vi "Set - Scalar - Complex.vi"(8 "error in":errorcluster, 9 "value":cdb, 10 "variable name":string, 11 "pipe in":T1) -> (0 "error out":errorcluster, 3 "pipe out":T1)   [LabVIEW 2013, in "GOLPI library.lvlib"]
uses:
  GOLPI library.lvlib
  LV Process.lvlibp/Pipe Handle.ctl
  Globals.vi
  LV Process.lvlibp
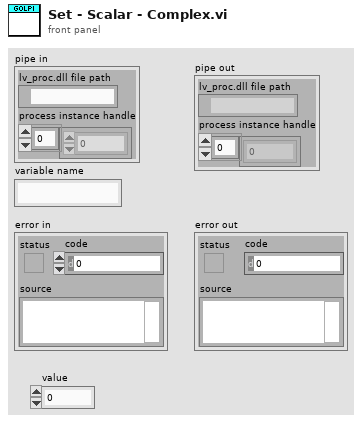
[diagram p1: front panel]
types:
  T1 = typedef "LV Process.lvlibp/Pipe Handle.ctl" = cluster{"lv_proc.dll file path":path, "process instance handle":u32[]}
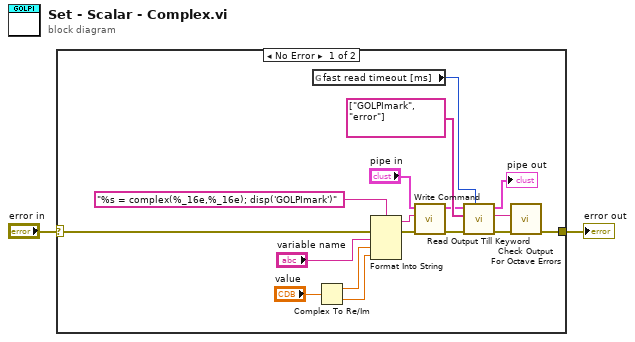
[diagram p0: block diagram]
diagram:
  n1 = case shown="No Error" "error in" {
    selector: "error in" -> [w17 w20]
    tunnel: [w6 w20] -> w2
    frame No Error {
      n2 = global read "Globals.vi" "fast read timeout [ms]"() -> (w8:u32)
      n3 = Complex To Re/Im(x + iy="value") -> (x=w4:dbl, y=w3:dbl)
      n4 = Format Into String(format string="%s = complex(%_16e,%_16e); disp('GOLPImark')", error in=w17, "variable name", w4, w3) -> (resulting string=w14:string, error out=w16:errorcluster)  [unwired: 1 in]
      n5 = call "Write Command.vi"("error in"=w16, "command"=w14, "pipe in"="pipe in") -> ("error out"=w13:errorcluster, "pipe out"=w10:T1)  [unwired: 7 in]
      n6 = call "Read Output Till Keyword.vi"("timeout [ms]"=w8, "error in"=w13, "keywords"=string[] ["GOLPImark", "error"], "pipe in"=w10) -> ("error out"=w12:errorcluster, "read buffer"=w9:string, "pipe out"=→"pipe out":T1)  [unwired: 4 in, 1 out]
      n7 = call "Check Output For Octave Errors.vi"("error in"=w12, "read buffer"=w9) -> ("error out"=w6:errorcluster)  [unwired: 9 in]
    }
    frame Error {
    }
  }
  "error out" <- w2
